vi "openConfigFile.vi"(8 "error in (no error)":errorcluster) -> (0 "error out":errorcluster, 3 "Path out":T1)   [LabVIEW 2018]
doc: "Open the default.ini file.\n\nNOTE: this is only for internal use. User does not call this function directly."
uses:
  <vilib>/Utility/config.llb/Config Data RefNum.ctl
  <vilib>/Utility/config.llb/NI_LVConfig.lvlib
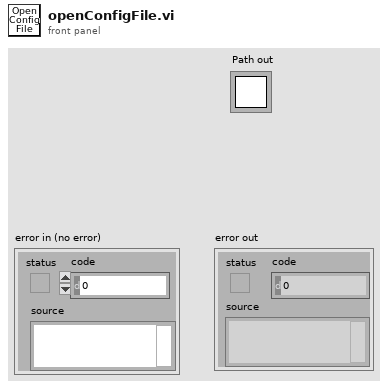
[diagram p1: front panel]
types:
  T1 = typedef "NI_LVConfig.lvlib/Config Data RefNum.ctl" = refnum<k1>
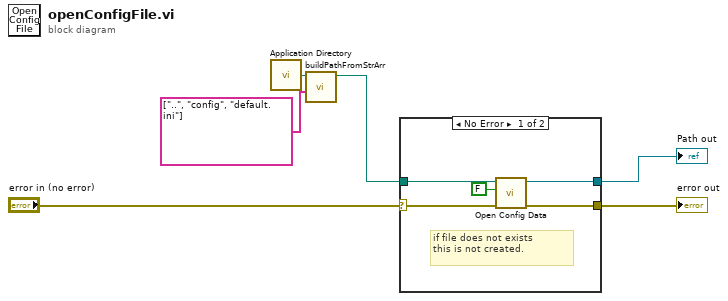
[diagram p0: block diagram]
diagram:
  n1 = call <vilib>:"Application Directory.vi"() -> ("Application Directory"=w5:path)
  n2 = call "buildPathFromStrArr.vi"("String Array"=string[] ["..", "config", "default.ini"], "Root Path"=w5) -> ("Absolute Path"=w3:path)  [unwired: 9 in]
  n3 = case shown="No Error" "error in (no error)" {
    selector: "error in (no error)" -> [w11 w12]
    tunnel: w3 -> [w10 _]
    tunnel: [w9 w12] -> w2
    tunnel: [w8 _] -> w1
    frame No Error {
      # "if file does not exists\nthis is not created."
      n4 = call <vilib>:"Open Config Data.vi"("error in (no error)"=w11, "create file if necessary (T)"=FALSE, "configuration file path"=w10) -> ("error out"=w9:errorcluster, "refnum"=w8:T1)  [unwired: 6 in, 1 out]
    }
    frame Error {
    }
  }
  "error out" <- w2
  "Path out" <- w1
